vi "test_SessionAlreadyCreated_CallCreateSessions_ReturnsError.vi"(8 "error in":errorcluster) -> (0 "error out":errorcluster, 2 "result":string, 3 "pass":bool)   [LabVIEW 2020, in "MeasurementServerTests.lvlib"]
uses:
  MeasurementServerTests.lvlib
  da6ffb6f-c1c9-4957-84dd-e9228483c454.vi
  ffc64c76-1568-41a3-8328-b9126ac9a28d.vi
  Helpers/Fake Instrument/Fake Instrument.lvclass
  \\tsclient\C/dev/measurementlink-labview/Source/Runtime/MeasurementLink Instrument/IInstrument/IInstrument.lvclass
  Runtime/MeasurementLink Measurement Server/Helpers/Error Strings Global Internal.vi
  Runtime/MeasurementLink Session Management/Session Reservation/Create Sessions Impl.vi
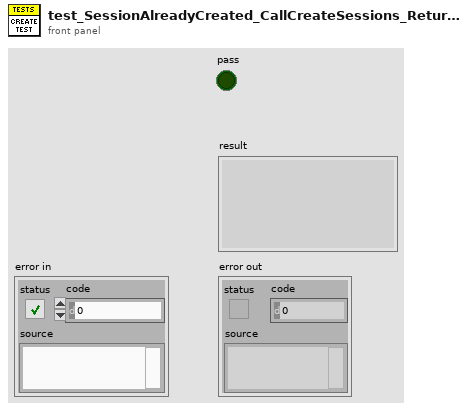
[diagram p1: front panel]
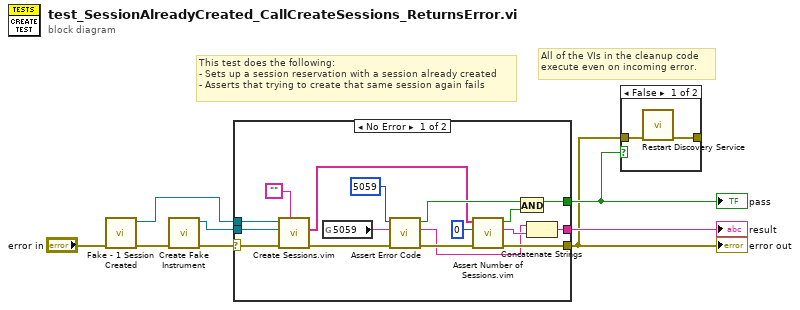
[diagram p0: block diagram]
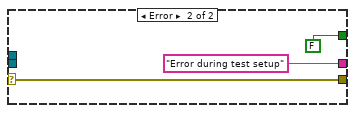
[diagram p2: hidden frame]
diagram:
  # "All of the VIs in the cleanup code\nexecute even on incoming error."
  # "This test does the following:\n- Sets up a session reservation with a session already created\n- Asserts that trying to create that same session again fails"
  n1 = call "Fake - 1 Session Created.vi"("error in"="error in") -> ("error out"=w2:errorcluster, "session reservation out"=w1:refnum<class "Session Reservation.lvclass">)  [unwired: 9 in]
  n2 = call "Create Fake Instrument.vi"("error in"=w2) -> ("error out"=w5:errorcluster, "fake instrument out"=w4:refnum<class "Fake Instrument.lvclass">)  [unwired: 9 in]
  n3 = case shown="No Error" w5 {
    selector: w5 -> [w23 w26]
    tunnel: [w14 w26] -> w6
    tunnel: [w13 FALSE] -> w7
    tunnel: [w11 "Error during test setup" ("f")] -> w8
    tunnel: w4 -> [w25 _]
    tunnel: w1 -> [w24 _]
    frame No Error {
      n4 = call "Create Sessions.vim"("session type"="", "error in"=w23, "instrument"=w25, "session reservation in"=w24) -> ("error out"=w22:errorcluster, "sessions"=w17:string[])  [unwired: 4 in, 2 out]
      n5 = global read "Error Strings Global Internal.vi" "5059"() -> (w18:string)
      n6 = call "Assert Error Code.vi"("error in"=w22, "expected error description"=w18, "expected error code"=5059) -> ("error out"=w15:errorcluster, "details"=w9:string, "error code match?"=w21:bool)  [unwired: 6 in]
      n7 = call "Assert Number of Sessions.vim"("error in"=w15, "expected number of sessions"=0, "sessions"=w17) -> ("error out"=w14:errorcluster, "result"=w10:string, "pass"=w12:bool)  [unwired: 6 in]
      n8 = And(x=w21, y=w12) -> (x .and. y?=w13:bool)
      n9 = Concatenate Strings(w9, w10) -> (w11:string)
    }
    frame Error {
    }
  }
  "error out" <- w6
  "pass" <- w7
  "result" <- w8
  n10 = case shown="False" w7 {
    tunnel: w6 -> [w30 _]
    tunnel: [w29 _] -> _
    frame False {
      n11 = call "Restart Discovery Service.vi"("error in"=w30) -> ("error out"=w29:errorcluster)  [unwired: 10 in]
    }
    frame True {
    }
  }
